vi "module.vi"(2 "jd":dbl, 3 "c":dbl, 4 "jb":dbl, 5 "a":dbl) -> (0 "Módulo fracionário":string, 1 "Módulo decimal":dbl)   [LabVIEW 2013]
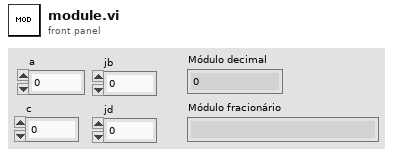
[diagram p1: front panel]
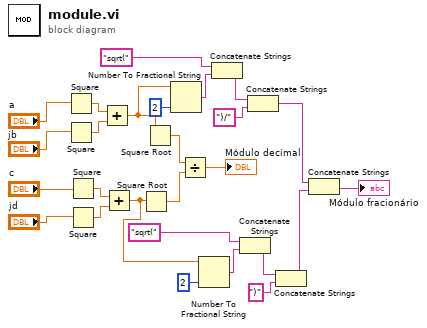
[diagram p0: block diagram]
diagram:
  n1 = Square(x="a") -> (x^2=w26:dbl)
  n2 = Square(x="jb") -> (x^2=w25:dbl)
  n3 = Square(x="c") -> (x^2=w24:dbl)
  n4 = Square(x="jd") -> (x^2=w23:dbl)
  n5 = Add(x=w26, y=w25) -> (x+y=w22:dbl)
  n6 = Add(x=w24, y=w23) -> (x+y=w11:dbl)
  n7 = Square Root(x=w11) -> (sqrt(x)=w16:dbl)
  n8 = Square Root(x=w22) -> (sqrt(x)=w17:dbl)
  n9 = Number To Fractional String(number=w22, precision (6)=i16 2) -> (F-format string=w20:string)  [unwired: 2 in]
  n10 = Divide(x=w17, y=w16) -> (x/y=→"Módulo decimal":dbl)
  n11 = Number To Fractional String(number=w11, precision (6)=i16 2) -> (F-format string=w13:string)  [unwired: 2 in]
  n12 = Concatenate Strings("sqrt(", w20) -> (w19:string)
  n13 = Concatenate Strings("sqrt(", w13) -> (w12:string)
  n14 = Concatenate Strings(w19, ")/") -> (w9:string)
  n15 = Concatenate Strings(w12, ")") -> (w8:string)
  n16 = Concatenate Strings(w9, w8) -> (→"Módulo fracionário":string)
